vi "LVClass_ComputePhaseSet Write ComputePhaseSet.vi"(8 "error in (no error)":errorcluster, 10 "ComputePhaseSet":T1, 11 "ComputePhaseSet in":refnum<class "ComputePhaseSet.lvclass">) -> (0 "error out":errorcluster, 3 "ComputePhaseSet out":refnum<class "ComputePhaseSet.lvclass">)   [LabVIEW 2020, in "ComputePhaseSet.lvclass"]
uses:
  ComputePhaseSet.lvclass
  Controls/ClassID.ctl
  Controls/Handle creation.ctl
  ComputePhaseSet.lvclass/ComputePhaseSet.ctl
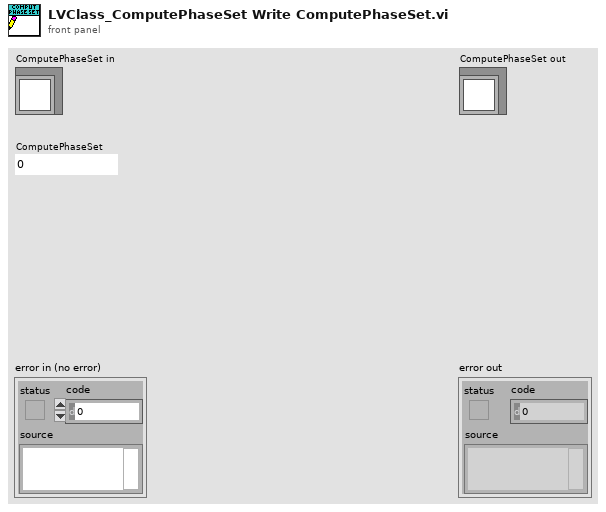
[diagram p1: front panel]
types:
  T1 = typedef "ClassID.ctl" = i64
  T2 = typedef "Handle creation.ctl" = enum16{"By ctor", "By write function"}
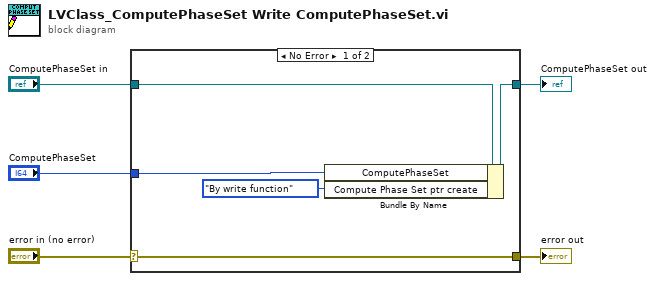
[diagram p0: block diagram]
diagram:
  n1 = case shown="No Error" "error in (no error)" {
    selector: "error in (no error)" -> [w10 w11]
    tunnel: [w10 w11] -> w4
    tunnel: [w8 w12] -> w2
    tunnel: "ComputePhaseSet in" -> [w9 w12]
    tunnel: "ComputePhaseSet" -> [w7 _]
    frame No Error {
      n2 = Bundle By Name(cluster=w9, "ComputePhaseSet"=w7, "Compute Phase Set ptr create"=Handle_creation."By write function") -> (w8:refnum<class "ComputePhaseSet.lvclass">)
    }
    frame Error {
    }
  }
  "error out" <- w4
  "ComputePhaseSet out" <- w2
